vi "DT2_discrete_a0.vi"(7 "D":dbl, 8 "error in (no error)":errorcluster, 9 "f0":dbl, 10 "Tcyc":dbl, 11 "TD":dbl) -> (0 "error out":errorcluster, 3 "a0":dbl)   [LabVIEW 2022 SP3]
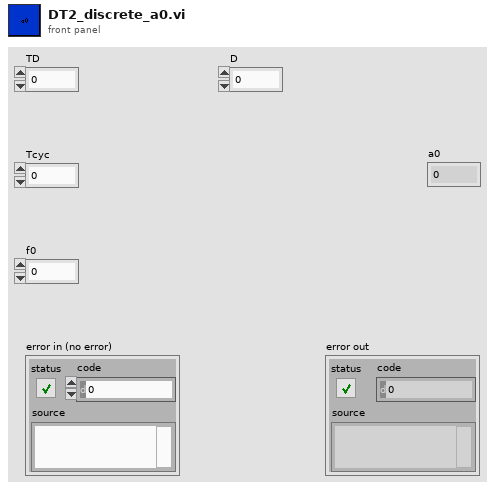
[diagram p1: front panel]
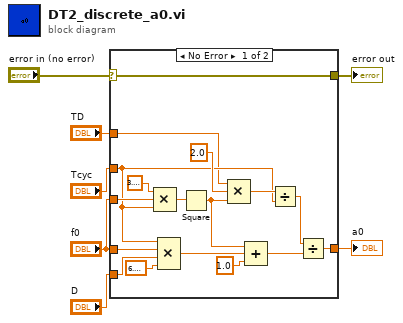
[diagram p0: block diagram]
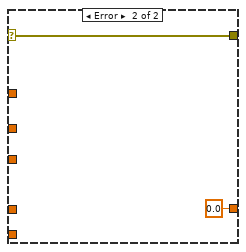
[diagram p2: hidden frame]
diagram:
  n1 = case shown="No Error" "error in (no error)" {
    selector: "error in (no error)" -> [w8 w25]
    tunnel: "f0" -> [w23 _]
    tunnel: "Tcyc" -> [w13 _]
    tunnel: "D" -> [w19 _]
    tunnel: "f0" -> [w18 _]
    tunnel: [w10 0.0] -> w5
    tunnel: "TD" -> [w9 _]
    tunnel: [w8 w25] -> w7
    frame No Error {
      n2 = Compound Arithmetic op=MULTIPLY(3.141592653589793, w23, w13) -> (w22:dbl)
      n3 = Compound Arithmetic op=MULTIPLY(w13, w18, w19, 6.283185307179586) -> (w16:dbl)
      n4 = Square(x=w22) -> (x^2=w17:dbl)
      n5 = Compound Arithmetic op=MULTIPLY(w9, 2.0 ("value"), w17) -> (w14:dbl)
      n6 = Compound Arithmetic op=ADD(w17, w16, 1.0 ("value")) -> (w11:dbl)
      n7 = Divide(x=w14, y=w13) -> (x/y=w12:dbl)
      n8 = Divide(x=w12, y=w11) -> (x/y=w10:dbl)
    }
    frame Error {
    }
  }
  "a0" <- w5
  "error out" <- w7
